vi "CreatePublicEvents.vi"(8 "error in (no error)":errorcluster, 11 "Inst.SPC":refnum<class "Inst.SPC.lvclass">) -> (0 "error out":errorcluster, 3 "Inst.SPC out":refnum<class "Inst.SPC.lvclass">)   [LabVIEW 2019, in "Inst.SPC.lvclass"]
doc: "---------------------------------------------------------------\nJKI State Machine Objects™\nhttp://jki.net/state-machine-objects/\nCopyright (C) 2005-2015, JKI <info@jki.net>\nALL RIGHTS RESERVEDJKI State Machine Objects (SMO) 1.0.0.4\nJKI - JKI\nCopyright (c) 2015, JKI"
uses:
  Inst.SPC.lvclass
  Typedefs/PublicEvents--Inst.SPC.MessageFromProcess.ctl
  <userlib>/LevyLab/Instrument Framework/SMOs/RemoteControl/Typedefs/Message--Cluster.ctl
  Inst.SPC.lvclass/Inst.SPC.ctl
  <userlib>/LevyLab/Instrument Framework/Instrument Types/VSource/Instrument.VSource.lvclass
  <userlib>/LevyLab/Instrument Framework/SMOs/RemoteControl/RemoteControl.lvclass
panel:
  # "For instructions on how to use the JKI State Machine Objects, examples and video tutorials, visit:\nhttp://jki.net/state-machine-objects/\n\nJKI State Machine Objects™\nhttp://jki.net/state-machine-objects/\nCopyright (C) 2005-2015, JKI <info@jki.net>\nALL RIGHTS RESERVED"
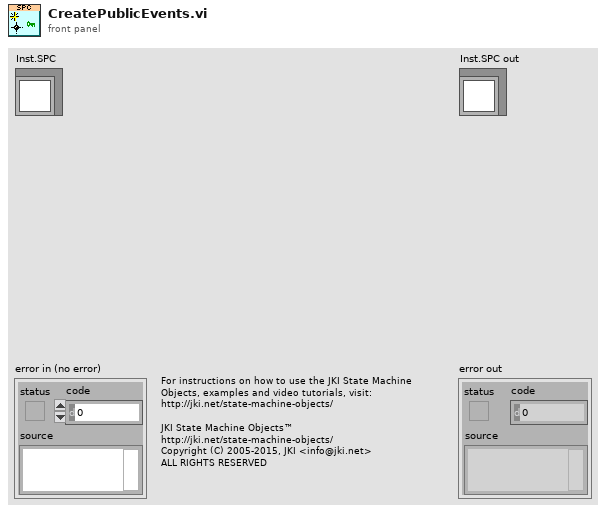
[diagram p1: front panel]
types:
  T1 = typedef "Inst.SPC.lvclass/PublicEvents--Inst.SPC.MessageFromProcess.ctl" = cluster{"Message":T2}
  T2 = typedef "RemoteControl.lvclass/Message--Cluster.ctl" = cluster{"Command":string, "Data":variant, "ID":string}
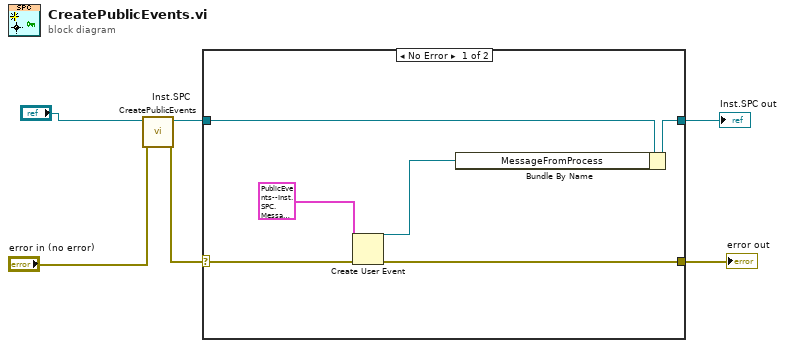
[diagram p0: block diagram]
diagram:
  n1 = call-parent "CreatePublicEvents.vi"("error in (no error)"="error in (no error)", "Instrument"="Inst.SPC") -> ("error out"=w3:errorcluster, "Instrument out"=w5:refnum<class "Inst.SPC.lvclass">)  [unwired: 8 in]
  n2 = case shown="No Error" w3 {
    selector: w3 -> [w11 w13]
    tunnel: w5 -> [w12 w14]
    tunnel: [w10 w13] -> w2
    tunnel: [w9 w14] -> w1
    frame No Error {
      n3 = Create User Event(user event datatype=T1 {"Message"={"Command"="", "Data"=variant(string ""), "ID"=""}} ("MessageToProcess"), error in=w11) -> (user event=w7:refnum<user-event>, error out=w10:errorcluster)
      n4 = Bundle By Name(cluster=w12, "MessageFromProcess"=w7) -> (w9:refnum<class "Inst.SPC.lvclass">)
    }
    frame Error {
    }
  }
  "error out" <- w2
  "Inst.SPC out" <- w1
